vi "GOOP_DrawWirePreview.vi"(1 "WireConfiguration":T1, 2 "Zoom":i32, 5 "Error in":errorcluster) -> (15 "Picture":picture, 19 "Error out":errorcluster)   [LabVIEW 2014]
uses:
  <resource>/Framework/Providers/Open_GDS/SubVIs/GOOP_WireConfigurationType.ctl
  <resource>/Framework/Providers/Open_GDS/SubVIs/GOOP_WirePattern.ctl
  <vilib>/picture/picture.llb/Draw True-Color Pixmap.vi
panel:
  in  "Wire":cluster{"x":i16, "y":i16}={"x"=40, "y"=54}
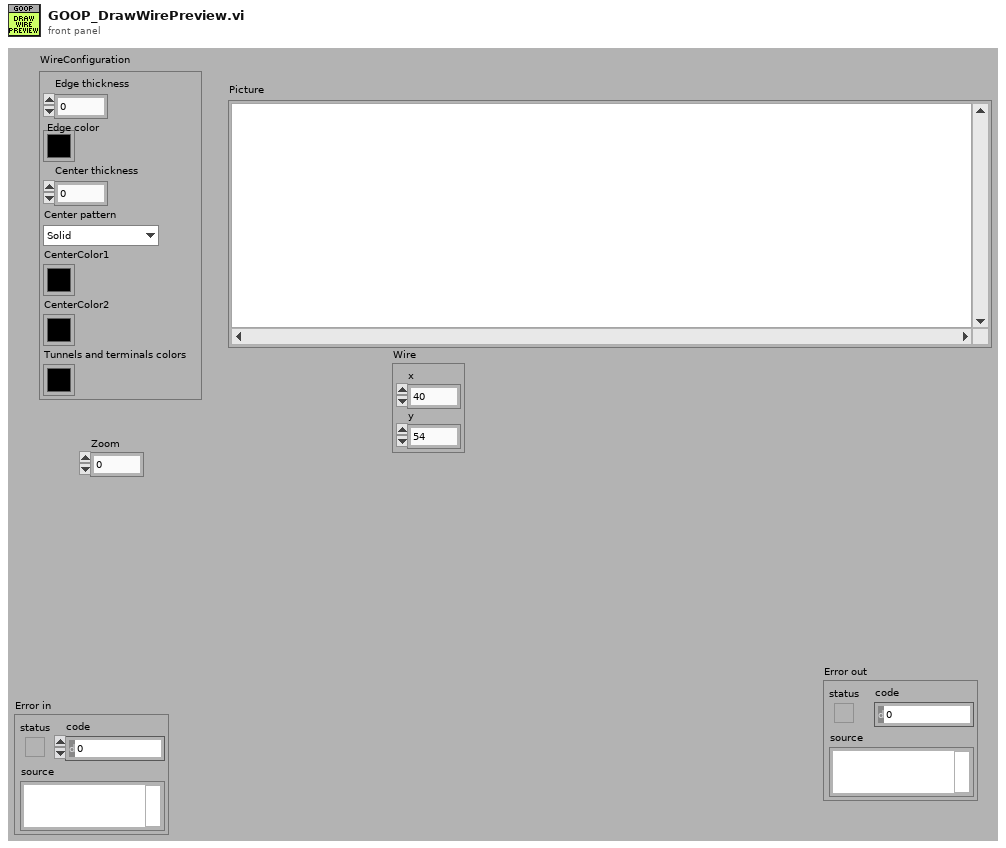
[diagram p1: front panel]
types:
  T1 = typedef "GOOP_WireConfigurationType.ctl" = cluster{"Edge thickness":i32, "Edge color":u32, "Center thickness":i32, "Center pattern":T2, "CenterColor1":u32, "CenterColor2":u32, "Tunnels and terminals colors":u32}
  T2 = typedef "GOOP_WirePattern.ctl" = enum16{"Solid", "Large dash", "Small dash"}
  T3 = cluster{"left":i16, "top":i16, "right":i16, "bottom":i16}
  T4 = typedef "imagedata.ctl" = cluster{"image type":i32, "image depth":i32, "image":u8[], "mask":u8[], "colors":u32[], "Rectangle":cluster{"left":i16, "top":i16, "right":i16, "bottom":i16}}
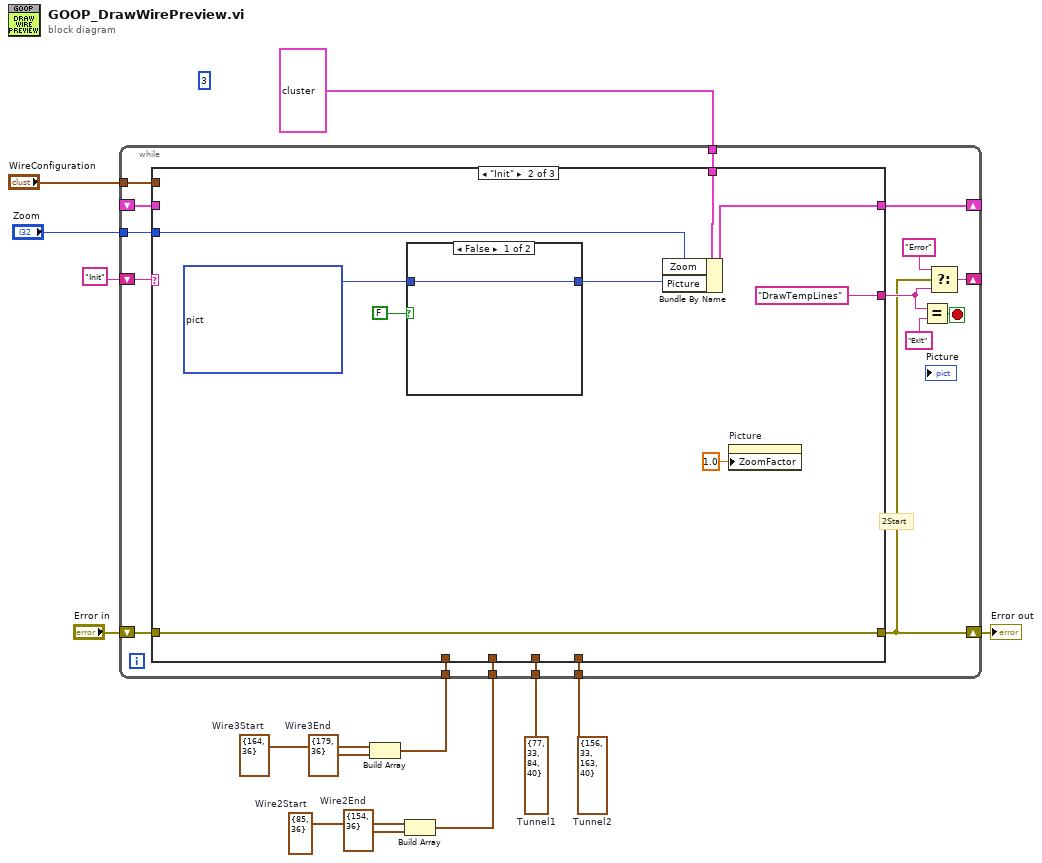
[diagram p0: block diagram]
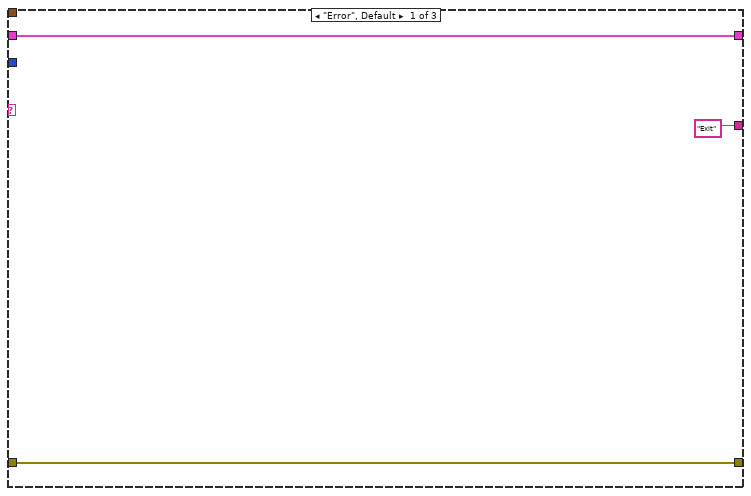
[diagram p2: hidden frame]
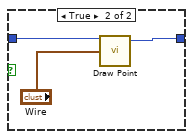
[diagram p3: hidden frame]
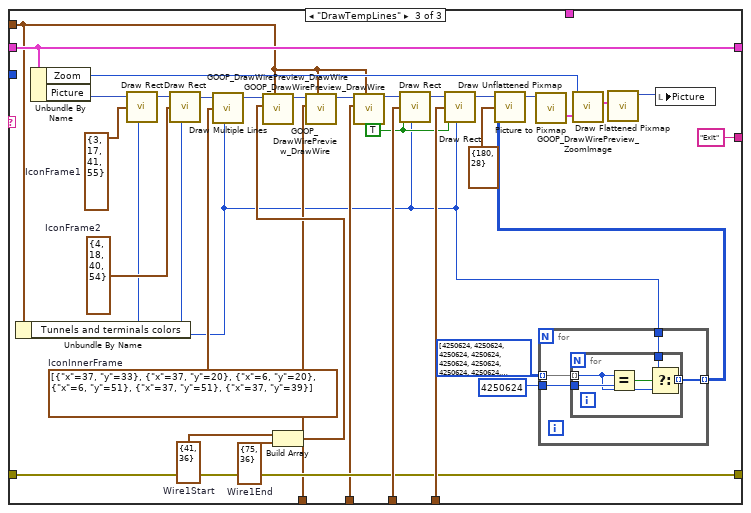
[diagram p4: hidden frame]
diagram:
  (unwired) i16 3 ("left")
  w5 = T3 {"left"=77, "top"=33, "right"=84, "bottom"=40}  # Tunnel1
  w4 = T3 {"left"=156, "top"=33, "right"=163, "bottom"=40}  # Tunnel2
  w10 = cluster{"x":i16, "y":i16} {"x"=179, "y"=36}  # Wire3End
  w11 = cluster{"x":i16, "y":i16} {"x"=164, "y"=36}  # Wire3Start
  w7 = cluster{"x":i16, "y":i16} {"x"=154, "y"=36}  # Wire2End
  w8 = cluster{"x":i16, "y":i16} {"x"=85, "y"=36}  # Wire2Start
  n1 = Build Array(w11, w10) -> (w9:cluster{"x":i16, "y":i16}[])
  n2 = Build Array(w8, w7) -> (w6:cluster{"x":i16, "y":i16}[])
  n3 = while {
    shift-right: [w24] -> w12
    shift-left: "Error in" -> [w31]
    shift-right: [w29] -> _
    shift-left: "Init" -> [w30]
    shift-right: [w23] -> _
    shift-left: _ -> [w22]
    tunnel: w9 -> [w21]
    tunnel: w6 -> [w20]
    tunnel: w5 -> [w19]
    tunnel: w4 -> [w18]
    tunnel: cluster{"Picture":picture, "Zoom":i32} {"Picture"=bytes[0], "Zoom"=3} -> [w17]
    tunnel: "WireConfiguration" -> [w16]
    tunnel: "Zoom" -> [w15]
    stop <- w28 stop-if-true
    n4 = case shown="\"Init\"" w30 {
      tunnel: w31 -> [w34 w42 w69]
      tunnel: [w34 w42 w69] -> w24
      tunnel: ["Exit" "DrawTempLines" "Exit"] -> w25
      tunnel: [w32 w41 w71] -> w23
      tunnel: w22 -> [w32 _ w71]
      tunnel: w21 -> [_ _ w52]
      tunnel: w20 -> [_ _ w51]
      tunnel: w19 -> [_ _ w73]
      tunnel: w18 -> [_ _ w72]
      tunnel: w17 -> [_ w38 _]
      tunnel: w16 -> [_ _ w49]
      tunnel: w15 -> [_ w36 _]
      frame "Error", Default {
      }
      frame "Init" {
        # "2Start"
        n5 = case shown="False" FALSE {
          tunnel: picture bytes[49464] ("new picture") -> [w44 w47]
          tunnel: [w44 w46] -> w39
          frame False {
          }
          frame True {
            n6 = call <vilib>:"Draw Point.vi"("picture"=w47, "point(x,y)"="Wire") -> ("new picture"=w46:picture)  [unwired: 7 in]
          }
        }
        n7 = Bundle By Name(cluster=w38, "Zoom"=w36, "Picture"=w39) -> (w41:cluster{"Picture":picture, "Zoom":i32})
        n8 = property on="Picture" class="Pict"("ZoomFactor"=sgl 1.0 ("Zoom Factor")) -> ()  [unwired: 2 in, 2 out]
      }
      frame "DrawTempLines" {
        w75 = cluster{"x":i16, "y":i16} {"x"=75, "y"=36}  # Wire1End
        w76 = cluster{"x":i16, "y":i16} {"x"=41, "y"=36}  # Wire1Start
        w78 = cluster{"x":i16, "y":i16}[] [{"x"=37, "y"=33}, {"x"=37, "y"=20}, {"x"=6, "y"=20}, {"x"=6, "y"=51}, {"x"=37, "y"=51}, {"x"=37, "y"=39}]  # IconInnerFrame
        w80 = T3 {"left"=4, "top"=18, "right"=40, "bottom"=54}  # IconFrame2
        w62 = T3 {"left"=3, "top"=17, "right"=41, "bottom"=55}  # IconFrame1
        w68 = TRUE ("fill?(F)")
        n9 = Unbundle By Name(w49) -> ("Tunnels and terminals colors"=w48:u32)
        n10 = Unbundle By Name(w71) -> ("Zoom"=w50:i32, "Picture"=w64:picture)
        n11 = call <vilib>:"Draw Rect.vi"("picture"=w64, "rect"=w62, "color(black)"=w48) -> ("new picture"=w81:picture)  [unwired: 6 in]
        n12 = call <vilib>:"Draw Rect.vi"("picture"=w81, "rect"=w80, "color(black)"=w48) -> ("new picture"=w79:picture)  [unwired: 6 in]
        n13 = call <vilib>:"Draw Multiple Lines.vi"("picture"=w79, "line endpoints"=w78, "color(black)"=w48) -> ("new picture"=w77:picture)  [unwired: 6 in]
        n14 = Build Array(w76, w75) -> (w74:cluster{"x":i16, "y":i16}[])
        n15 = call <resource>:"GOOP_DrawWirePreview_DrawWire.vi"("WireConfiguration"=w49, "Array"=w74, "PictureIn"=w77) -> ("PictureOut"=w55:picture)  [unwired: 8 in]
        n16 = call <resource>:"GOOP_DrawWirePreview_DrawWire.vi"("WireConfiguration"=w49, "Array"=w52, "PictureIn"=w55) -> ("PictureOut"=w53:picture)  [unwired: 8 in]
        n17 = call <resource>:"GOOP_DrawWirePreview_DrawWire.vi"("WireConfiguration"=w49, "Array"=w51, "PictureIn"=w53) -> ("PictureOut"=w54:picture)  [unwired: 8 in]
        n18 = call <vilib>:"Draw Rect.vi"("picture"=w54, "rect"=w73, "fill?(F)"=w68, "color(black)"=w48) -> ("new picture"=w63:picture)  [unwired: 5 in]
        n19 = call <vilib>:"Draw Rect.vi"("picture"=w63, "rect"=w72, "fill?(F)"=w68, "color(black)"=w48) -> ("new picture"=w58:picture)  [unwired: 5 in]
        n20 = for {
          tunnel: u32[][] [[4250624, 4250624, 4250624, 4250624, 4250624, 4250624, 4250624, 4250624, 4250624, 4250624, 4250624, 4250624, 4250624, 4250624, 4250624, 4250624, 4250624, 4250624, 4250624, 4250624, 4250624, 4250624, 4250624, 4250624, 4250624, 4250624, 4250624, 4250624, 4250624, 4250624, 4250624, 4250624], [4250624, 16777215, 16777215, 16777215, 16777215, 16777215, 16777215, 16777215, 16777215, 16777215, 16777215, 16777215, 16777215, 16777215, 16777215, 16777215, 16777215, 16777215, 16777215, 16777215, 16777215, 16777215, 16777215, 16777215, 16777215, 16777215, 16777215, 16777215, 16777215, 16777215, 16777215, 4250624], [4250624, 16777215, 16777215, 16777215, 16777215, 16777215, 16777215, 16777215, 16777215, 16777215, 16777215, 16777215, 16777215, 16777215, 16777215, 16777215, 16777215, 16777215, 16777215, 16777215, 16777215, 16777215, 16777215, 16777215, 16777215, 16777215, 16777215, 16777215, 16777215, 16777215, 16777215, 4250624], [4250624, 16777215, 16777215, 4250624, 4250624, 4250624, 4250624, 4250624, 4250624, 4250624, 4250624, 4250624, 4250624, 4250624, 4250624, 4250624, 4250624, 4250624, 4250624, 4250624, 4250624, 4250624, 4250624, 4250624, 4250624, 4250624, 4250624, 4250624, 4250624, 16777215, 16777215, 4250624], [4250624, 16777215, 16777215, 4250624, 16777215, 16777215, 16777215, 16777215, 16777215, 16777215, 16777215, 16777215, 16777215, 16777215, 16777215, 16777215, 16777215, 16777215, 16777215, 16777215, 16777215, 16777215, 16777215, 16777215, 16777215, 16777215, 16777215, 16777215, 4250624, 16777215, 16777215, 4250624], [4250624, 16777215, 16777215, 4250624, 0, 16777215, 16777215, 16777215, 16777215, 4250624, 4250624, 4250624, 16777215, 16777215, 4250624, 4250624, 4250624, 4250624, 16777215, 16777215, 16777215, 16777215, 4250624, 4250624, 16777215, 16777215, 16777215, 16777215, 4250624, 16777215, 16777215, 4250624], [4250624, 16777215, 16777215, 4250624, 0, 0, 16777215, 16777215, 4250624, 4250624, 16777215, 4250624, 4250624, 16777215, 4250624, 4250624, 16777215, 4250624, 4250624, 16777215, 16777215, 16777215, 4250624, 4250624, 16777215, 16777215, 16777215, 16777215, 4250624, 16777215, 16777215, 4250624], [4250624, 16777215, 16777215, 4250624, 0, 0, 0, 16777215, 4250624, 4250624, 16777215, 4250624, 4250624, 16777215, 4250624, 4250624, 4250624, 4250624, 16777215, 16777215, 16777215, 16777215, 4250624, 4250624, 16777215, 16777215, 16777215, 16777215, 4250624, 16777215, 16777215, 4250624], [4250624, 16777215, 16777215, 4250624, 0, 0, 0, 16777215, 4250624, 4250624, 16777215, 4250624, 4250624, 16777215, 4250624, 4250624, 16777215, 4250624, 4250624, 16777215, 4250624, 16777215, 4250624, 4250624, 16777215, 16777215, 16777215, 16777215, 4250624, 16777215, 16777215, 4250624], [4250624, 16777215, 16777215, 4250624, 0, 0, 16777215, 16777215, 4250624, 4250624, 16777215, 4250624, 4250624, 16777215, 4250624, 4250624, 16777215, 4250624, 4250624, 16777215, 4250624, 16777215, 4250624, 4250624, 16777215, 16777215, 16777215, 16777215, 4250624, 16777215, 16777215, 4250624], [4250624, 16777215, 16777215, 4250624, 0, 16777215, 16777215, 16777215, 16777215, 4250624, 4250624, 4250624, 16777215, 16777215, 4250624, 4250624, 4250624, 4250624, 16777215, 16777215, 16777215, 4250624, 4250624, 16777215, 16777215, 16777215, 16777215, 16777215, 4250624, 16777215, 16777215, 4250624], [4250624, 16777215, 16777215, 4250624, 16777215, 16777215, 16777215, 16777215, 16777215, 16777215, 16777215, 16777215, 16777215, 16777215, 16777215, 16777215, 16777215, 16777215, 16777215, 16777215, 16777215, 16777215, 16777215, 16777215, 16777215, 16777215, 16777215, 16777215, 4250624, 16777215, 16777215, 4250624], [4250624, 16777215, 16777215, 4250624, 4250624, 4250624, 4250624, 4250624, 4250624, 4250624, 4250624, 4250624, 4250624, 4250624, 4250624, 4250624, 4250624, 4250624, 4250624, 4250624, 4250624, 4250624, 4250624, 4250624, 4250624, 4250624, 4250624, 4250624, 4250624, 16777215, 16777215, 4250624], [4250624, 16777215, 16777215, 16777215, 16777215, 16777215, 16777215, 16777215, 16777215, 16777215, 16777215, 16777215, 16777215, 16777215, 16777215, 16777215, 16777215, 16777215, 16777215, 16777215, 16777215, 16777215, 16777215, 16777215, 16777215, 16777215, 16777215, 16777215, 16777215, 16777215, 16777215, 4250624], [4250624, 16777215, 16777215, 16777215, 16777215, 16777215, 16777215, 16777215, 16777215, 16777215, 16777215, 16777215, 16777215, 16777215, 16777215, 16777215, 16777215, 16777215, 16777215, 16777215, 16777215, 16777215, 16777215, 16777215, 16777215, 16777215, 16777215, 16777215, 16777215, 16777215, 16777215, 4250624], [4250624, 4250624, 4250624, 4250624, 4250624, 4250624, 4250624, 4250624, 4250624, 4250624, 4250624, 4250624, 4250624, 4250624, 4250624, 4250624, 4250624, 4250624, 4250624, 4250624, 4250624, 4250624, 4250624, 4250624, 4250624, 4250624, 4250624, 4250624, 4250624, 4250624, 4250624, 4250624]] ("24-bit pixmap") -> [w85] mode=indexing
          tunnel: u32 4250624 -> [w84]
          tunnel: [w83] -> w56 mode=indexing
          tunnel: w48 -> [w82]
          n21 = for {
            tunnel: w85 -> [w88] mode=indexing
            tunnel: w84 -> [w90]
            tunnel: [w87] -> w83 mode=indexing
            tunnel: w82 -> [w86]
            n22 = Equal?(x=w88, y=w90) -> (x = y?=w89:bool)
            n23 = Select(t=w86, s=w89, f=w88) -> (s? t:f=w87:u32)
          }
        }
        n24 = call-poly <vilib>:"Draw Unflattened Pixmap.vi"("picture"=w58, "top left point(0, 0)"=cluster{"x":i16, "y":i16} {"x"=180, "y"=28}, "data (RGB format)"=w56) -> ("new picture"=w57:picture)  [unwired: 6 in]
        n25 = call <vilib>:"Picture to Pixmap.vi"("picture"=w57) -> ("image data"=w67:T4)  [unwired: 9 in, 1 out]
        n26 = call <resource>:"GOOP_DrawWirePreview_ZoomImage.vi"("image data 2"=w67, "Zoom"=w50) -> ("image data"=w66:T4)
        n27 = call <vilib>:"Draw Flattened Pixmap.vi"("image data"=w66) -> ("new picture"=w65:picture)  [unwired: 8 in]
        n28 = local write "Picture"(w65) -> ()
      }
    }
    n29 = Equal?(x=w25, y="Exit") -> (x = y?=w28:bool)
    n30 = Select(t="Error", s=w24, f=w25) -> (s? t:f=w29:string)
  }
  "Error out" <- w12
